vi "RecordIntoDB.vi"(6 "Debug":bool, 7 "Model":string, 8 "error in":errorcluster caption="错误输入", 9 "Time":string, 10 "产品类别":refnum<vi>, 11 "ArrayIn":string[](array[string])) -> (0 "error out":errorcluster caption="错误输出", 3 "Result":string)   [LabVIEW 2013]
panel:
  in  "产品类":u16(ring) caption="产品类别" items=["带卡产品", "非带卡产品"]
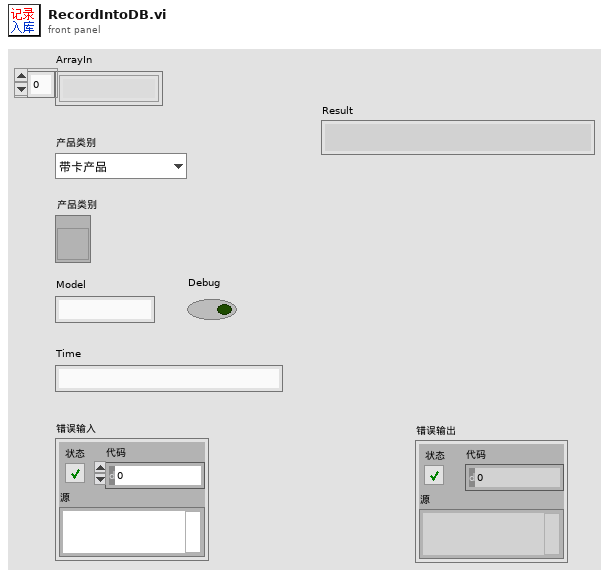
[diagram p1: front panel]
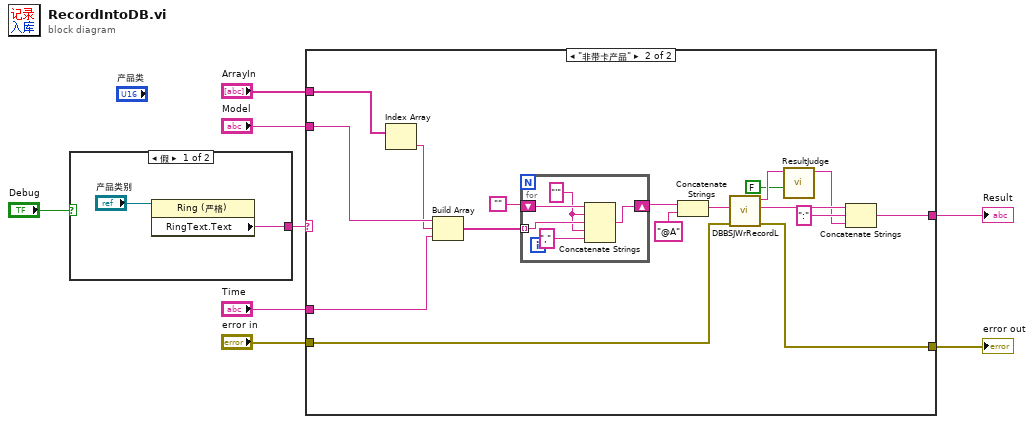
[diagram p0: block diagram]
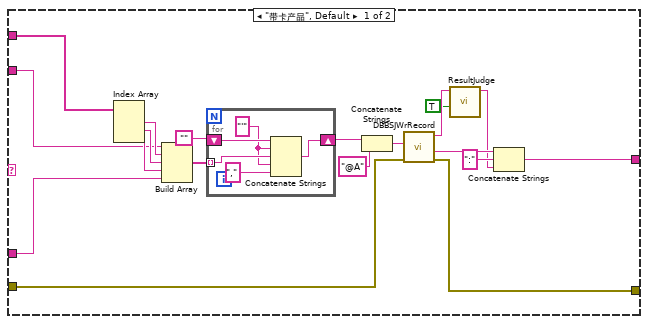
[diagram p2: hidden frame]
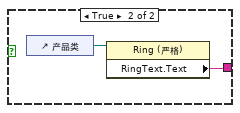
[diagram p3: hidden frame]
diagram:
  n1 = case shown="假" "Debug" {
    tunnel: [w9 w11] -> w7
    frame False {
      n2 = property class="Ring (严格)"(reference="产品类别") -> ("RingText.Text"=w9:string)  [unwired: 1 in, 2 out]
    }
    frame True {
      n3 = control-ref of="产品类"() -> (w12:refnum<vi>)
      n4 = property class="Ring (严格)"(reference=w12) -> ("RingText.Text"=w11:string)  [unwired: 1 in, 2 out]
    }
  }
  n5 = case shown="\"非带卡产品\"" w7 {
    tunnel: "ArrayIn" -> [w19 w53]
    tunnel: "Model" -> [w18 w51]
    tunnel: "Time" -> [w17 w49]
    tunnel: "error in" -> [w16 w44]
    tunnel: [w15 w38] -> w2
    tunnel: [w14 w39] -> w1
    frame "带卡产品", Default {
      n6 = Index Array(array=w19) -> (element #1=w30:string, element #2=w29:string, element #3=w28:string)  [unwired: 3 in]
      n7 = Build Array(w18, w30, w29, w28, w17) -> (w27:string[])
      n8 = for {
        tunnel: w27 -> [w35] mode=indexing
        shift-right: [w32] -> w25
        shift-left: "" -> [w36]
        w34 = "'" ("字符串")
        n9 = Concatenate Strings(w36, w34, w35, w34, "," ("字符串")) -> (w32:string)
      }
      n10 = Concatenate Strings(w25, "@A" ("字符串")) -> (w24:string)
      n11 = call "DBBSJWrRecord.vi"("error in"=w16, "String"=w24) -> ("error out"=w15:errorcluster, "SN"=w23:string, "ReportStr"=w21:string)  [unwired: 5 in, 2 out]
      n12 = call "ResultJudge.vi"("带卡？"=TRUE, "StrIn"=w21) -> ("StrOut"=w20:string)  [unwired: 8 in, 1 out]
      n13 = Concatenate Strings(w23, ":" ("字符串"), w20) -> (w14:string)
    }
    frame "非带卡产品" {
      n14 = Index Array(array=w53) -> (element=w50:string)  [unwired: 1 in]
      n15 = Build Array(w51, w50, w49) -> (w48:string[])
      n16 = for {
        tunnel: w48 -> [w57] mode=indexing
        shift-right: [w54] -> w47
        shift-left: "" -> [w58]
        w56 = "'" ("字符串")
        n17 = Concatenate Strings(w58, w56, w57, w56, "," ("字符串")) -> (w54:string)
      }
      n18 = Concatenate Strings(w47, "@A" ("字符串")) -> (w45:string)
      n19 = call "DBBSJWrRecordL.vi"("error in"=w44, "String"=w45) -> ("error out"=w38:errorcluster, "SN"=w41:string, "ReportStr"=w43:string)  [unwired: 6 in, 1 out]
      n20 = call "ResultJudge.vi"("带卡？"=FALSE, "StrIn"=w43) -> ("StrOut"=w40:string)  [unwired: 8 in, 1 out]
      n21 = Concatenate Strings(w41, ":" ("字符串"), w40) -> (w39:string)
    }
  }
  "error out" <- w2
  "Result" <- w1
